vi "셔플.vi"() -> ()   [LabVIEW 2020]
uses:
  <vilib>/Utility/file.llb/Read Delimited Spreadsheet (DBL).vi
  <vilib>/Utility/file.llb/Write Delimited Spreadsheet (DBL).vi
panel:
  out "배열":dbl[](array[numeric])
  out "all rows":dbl[][](array[numeric]) caption="모든 행"
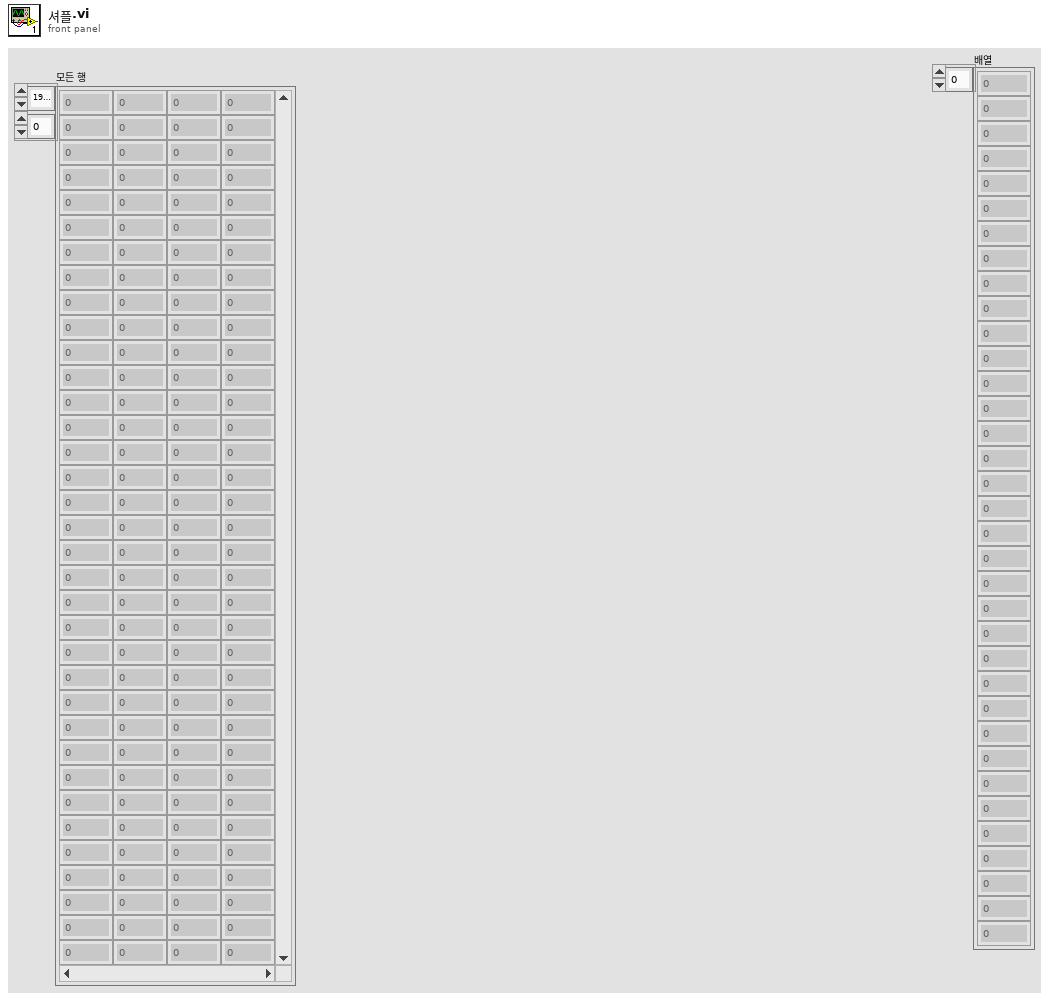
[diagram p1: front panel]
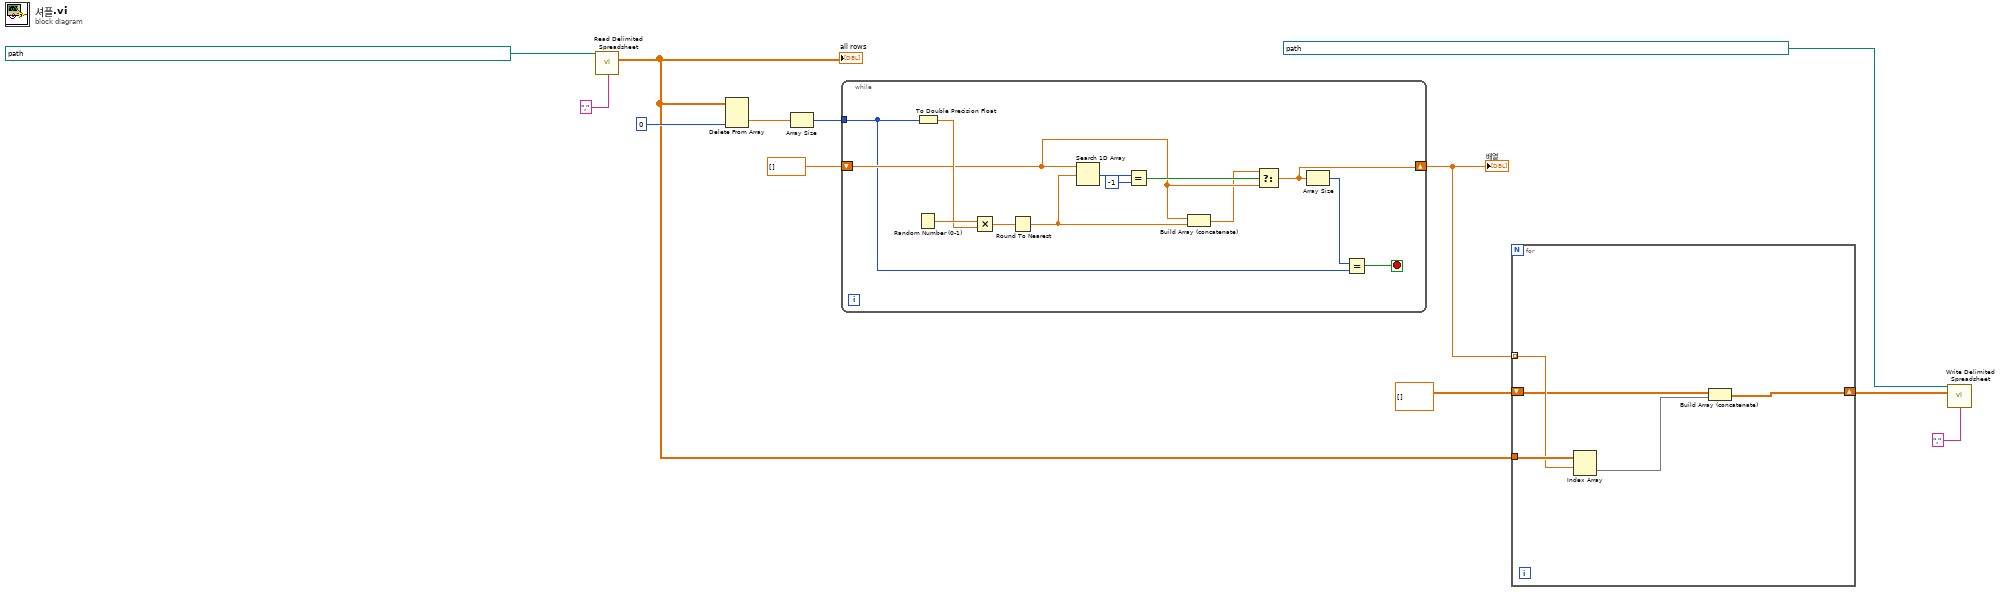
[diagram p0: block diagram]
diagram:
  n1 = call-poly <vilib>:"Read Delimited Spreadsheet.vi"("file path (dialog if empty)"=path "C:/Users/User/Desktop/이덕규/LabVIEW/교육/2022/2022.03.24~2022.03.25 대한상공회의소/Python/test/Test4.csv", "delimiter (\\t)"="," ("delimiter (\\t)")) -> ("all rows"=w5:dbl[][])  [unwired: 8 in, 5 out]
  "all rows" <- w5
  n2 = Delete From Array(array=w5, index (col)=0 ("비활성화된 인덱스 (열)")) -> (deleted portion=w9:dbl[])  [unwired: 2 in, 1 out]
  n3 = Array Size(array=w9) -> (size(s)=w8:i32)
  n4 = while {
    tunnel: w8 -> [w14]
    shift-right: [w16] -> w6
    shift-left: dbl[] [] -> [w19]
    stop <- w13 stop-if-true
    n5 = Random Number (0-1)() -> (number: 0 to 1=w25:dbl)
    n6 = To Double Precision Float(number=w14) -> (double precision float=w24:dbl)
    n7 = Multiply(x=w25, y=w24) -> (x*y=w23:dbl)
    n8 = Round To Nearest(number=w23) -> (nearest integer value=w18:dbl)
    n9 = Search 1D Array(1D array=w19, element=w18) -> (index of element=w22:i32)  [unwired: 1 in]
    n10 = Equal?(x=w22, y=-1) -> (x = y?=w20:bool)
    n11 = Build Array (concatenate)(w19, w18) -> (w17:dbl[])
    n12 = Select(t=w17, s=w20, f=w19) -> (s? t:f=w16:dbl[])
    n13 = Array Size(array=w16) -> (size(s)=w15:i32)
    n14 = Equal?(x=w15, y=w14) -> (x = y?=w13:bool)
  }
  "배열" <- w6
  n15 = for {
    tunnel: w6 -> [w29] mode=indexing
    tunnel: w5 -> [w30]
    shift-right: [w26] -> w2
    shift-left: dbl[][] [] -> [w28]
    n16 = Index Array(array=w30, index (row)=w29) -> (element=w27:dbl[])  [unwired: 1 in]
    n17 = Build Array (concatenate)(w28, w27) -> (w26:dbl[][])
  }
  n18 = call-poly <vilib>:"Write Delimited Spreadsheet.vi"("file path (dialog if empty)"=path "C:/Users/User/Desktop/이덕규/LabVIEW/교육/2022/2022.03.24~2022.03.25 대한상공회의소/Python/test/Test4.csv", "2D data"=w2, "delimiter (\\t)"="," ("delimiter (\\t)")) -> ()  [unwired: 11 in, 2 out]
